vi "UserEvents-init.vi"(2 "entrée d'erreur (pas d'erreur)":errorcluster) -> (0 "sortie d'erreur":errorcluster, 1 "Controls":T1)   [LabVIEW 2015]
uses:
  Classes/Experiment.lvclass
  controls/Controls.ctl
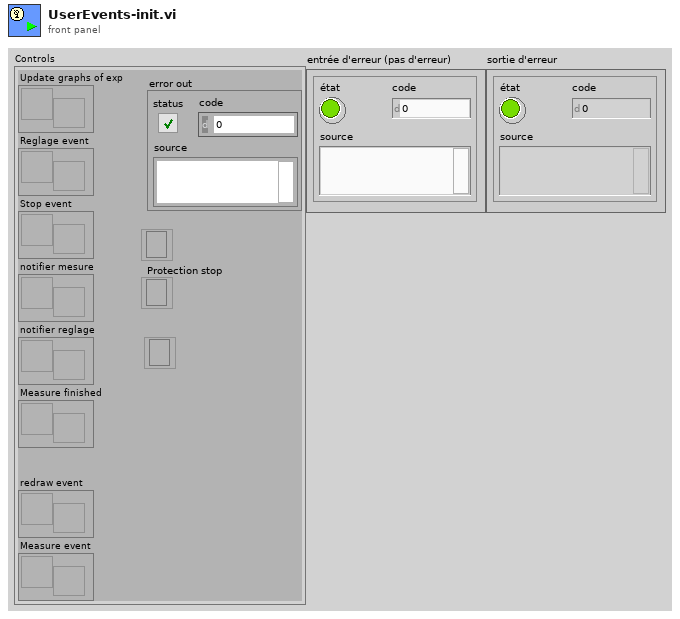
[diagram p1: front panel]
types:
  T1 = typedef "Controls.ctl" = cluster{"Update graphs of exp":refnum<user-event>, "Reglage event":refnum<user-event>, "Stop event":refnum<user-event>, "notifier mesure":refnum<notifier>, "notifier reglage":refnum<notifier>, "Measure finished":refnum<user-event>, "control registration ref":refnum<event-registration>, "redraw event":refnum<user-event>, "Measure event":refnum<user-event>, "Mes, Reg, Stop Registration ref":refnum<event-registration>, "error out":errorcluster, "Protection stop":refnum<event-registration>}
  T2 = cluster{"Operate":bool, "Experiment":refnum<class "Experiment.lvclass">, "group path":path}
  T3 = cluster{"Operate":bool, "Experiment":refnum<class "Experiment.lvclass">}
  T4 = cluster{"Full/Part":bool, "Item names":string[], "Exp number":i32}
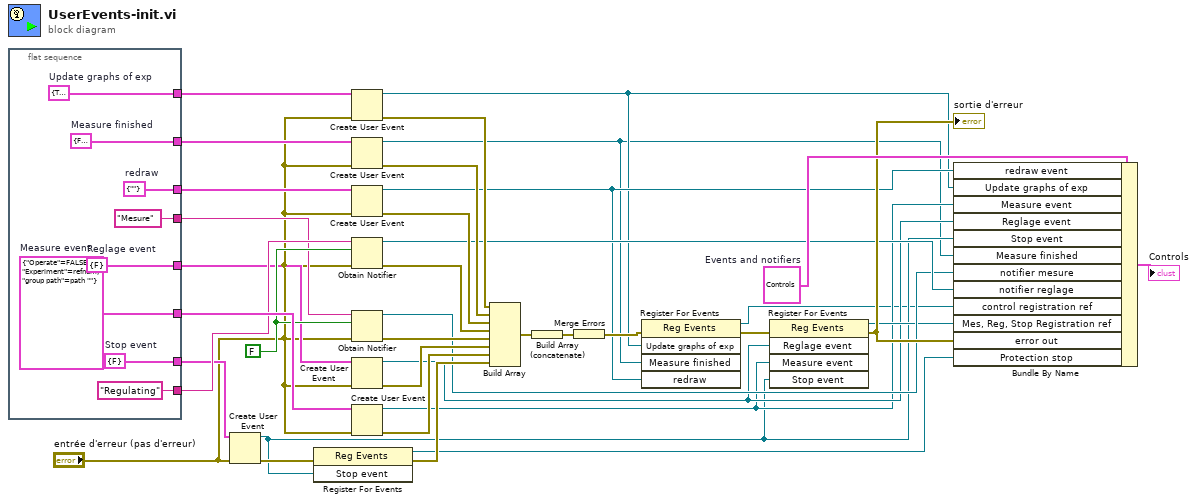
[diagram p0: block diagram]
diagram:
  w14 = T1 {"Update graphs of exp"=refnum, "Reglage event"=refnum, "Stop event"=refnum, "notifier mesure"=refnum, "notifier reglage"=refnum, "Measure finished"=refnum, "control registration ref"=refnum, "redraw event"=refnum, "Measure event"=refnum, "Mes, Reg, Stop Registration ref"=refnum, "error out"={"status"=FALSE, "code"=0, "source"=""}, "Protection stop"=refnum}  # Events and notifiers
  w24 = FALSE
  n1 = flat-sequence {
    tunnel: [w45] -> w16
    tunnel: [w44] -> w17
    tunnel: [w43] -> w18
    tunnel: ["Mesure" ("name (unnamed)")] -> w19
    tunnel: ["Regulating" ("name (unnamed)")] -> w20
    tunnel: [w40] -> w25
    tunnel: [w39] -> w26
    tunnel: [w38] -> w27
    frame #0 {
      w38 = T2 {"Operate"=FALSE, "Experiment"=refnum, "group path"=path ""}  # Measure event
      w39 = cluster{"what to redraw":string} {"what to redraw"=""}  # redraw
      w40 = T3 {"Operate"=FALSE, "Experiment"=refnum}  # Measure finished
      w44 = cluster{"Stop":bool} {"Stop"=FALSE}  # Stop event
      w45 = T4 {"Full/Part"=TRUE, "Item names"=[], "Exp number"=0}  # Update graphs of exp
      w43 = cluster{"Operate":bool} {"Operate"=FALSE}  # Reglage event
    }
  }
  n2 = Create User Event(user event datatype=w17, error in="entrée d'erreur (pas d'erreur)") -> (user event=w7:refnum<user-event>, error out=w36:errorcluster)
  n3 = register-events(error in=w36, w7) -> (reference out=w2:refnum<event-registration>, error out=w37:errorcluster)  [unwired: 1 in]
  n4 = Create User Event(user event datatype=w16, error in="entrée d'erreur (pas d'erreur)") -> (user event=w5:refnum<user-event>, error out=w31:errorcluster)
  n5 = Create User Event(user event datatype=w25, error in="entrée d'erreur (pas d'erreur)") -> (user event=w4:refnum<user-event>, error out=w32:errorcluster)
  n6 = Create User Event(user event datatype=w26, error in="entrée d'erreur (pas d'erreur)") -> (user event=w6:refnum<user-event>, error out=w33:errorcluster)
  n7 = Obtain Notifier(name (unnamed)=w20, notification data type=w24, error in (no error)="entrée d'erreur (pas d'erreur)") -> (notifier out=w12:refnum<notifier>, error out=w22:errorcluster)  [unwired: 1 in, 1 out]
  n8 = Obtain Notifier(name (unnamed)=w19, notification data type=w24, error in (no error)="entrée d'erreur (pas d'erreur)") -> (notifier out=w11:refnum<notifier>, error out=w23:errorcluster)  [unwired: 1 in, 1 out]
  n9 = Create User Event(user event datatype=w18, error in="entrée d'erreur (pas d'erreur)") -> (user event=w9:refnum<user-event>, error out=w21:errorcluster)
  n10 = Create User Event(user event datatype=w27, error in="entrée d'erreur (pas d'erreur)") -> (user event=w8:refnum<user-event>, error out=w28:errorcluster)
  n11 = Build Array(w31, w32, w33, w22, w23, w21, w28, w37) -> (w29:errorcluster[])
  n12 = Build Array (concatenate)(w29) -> (w30:errorcluster[])
  n13 = Merge Errors(w30) -> (w34:errorcluster)
  n14 = register-events(error in=w34, w5, w4, w6) -> (reference out=w1:refnum<event-registration>, error out=w35:errorcluster)  [unwired: 1 in]
  n15 = register-events(error in=w35, w9, w8, w7) -> (reference out=w10:refnum<event-registration>, error out=w13:errorcluster)  [unwired: 1 in]
  "sortie d'erreur" <- w13
  n16 = Bundle By Name(cluster=w14, "redraw event"=w6, "Update graphs of exp"=w5, "Measure event"=w8, "Reglage event"=w9, "Stop event"=w7, "Measure finished"=w4, "notifier mesure"=w11, "notifier reglage"=w12, "control registration ref"=w1, "Mes, Reg, Stop Registration ref"=w10, "error out"=w13, "Protection stop"=w2) -> (→"Controls":T1)
